vi "Задание_АБ_система ask.vi"() -> ()   [LabVIEW 2017]
uses:
  <vilib>/Analysis/baseanly.llb/Mean (DBL).vi
  <vilib>/gmath/statdist.llb/Normal Random.vi
  <vilib>/Analysis/3filter.llb/Bessel Filter (DBL).vi
  <vilib>/Analysis/NI_AALBase.lvlib
  <vilib>/gmath/NI_Gmath.lvlib
panel:
  out "subarray":dbl[](array[numeric])
  out "Декодированное сообщение 2":dbl[](array[numeric])
  out "x*y 2":i32
  out "x*y":i32
  out "size(s) 2":i32[](array[numeric])
  out "Размер окна с паузами":i32
  out "size(s)":i32
  out "output array":dbl[](array[numeric])
  out "Декодированное сообщение":dbl[](array[numeric])
  in  "Кол-во копий":i32=5
  out "Подготовленный к отправке мажоритарный код":dbl[][](array[numeric])
  out "0, 1":i16[](array[numeric])
  in  "Пороговое значение 2":dbl
  out "Среднее значение":dbl[](array[numeric])
  out "Шум на основе распределения Рэлея":dbl[](graph)
  out "Демодулированный и отфильтрованный сигнал":dbl[](graph)
  in  "Нижняя частота среза":dbl
  in  "Порядок фильтра":i64(slide) scale=0.0..20.0
  in  "Переменная floor(x/y)":i32
  out "Модулирующий сигнал":dbl[](graph)
  out "Частотно модулированный цифровой сигнал":dbl[](graph)
  in  "см. 1.2 Циклов в секунду":i32(slide) scale=4.0..50.0
  in  "Сколько битов брать":i32=4
  out "Радио сигнал с паузами":dbl[](graph)
  in  "Кол-во выборок":i32=400
  out "Массив с паузами":dbl[](array[numeric])
  in  "Количество бит":i32=8
  out "Вырезка из массива":dbl[](array[numeric])
  out "Биты на выходе 1":dbl[](array[numeric])
  # "Демодуляция"
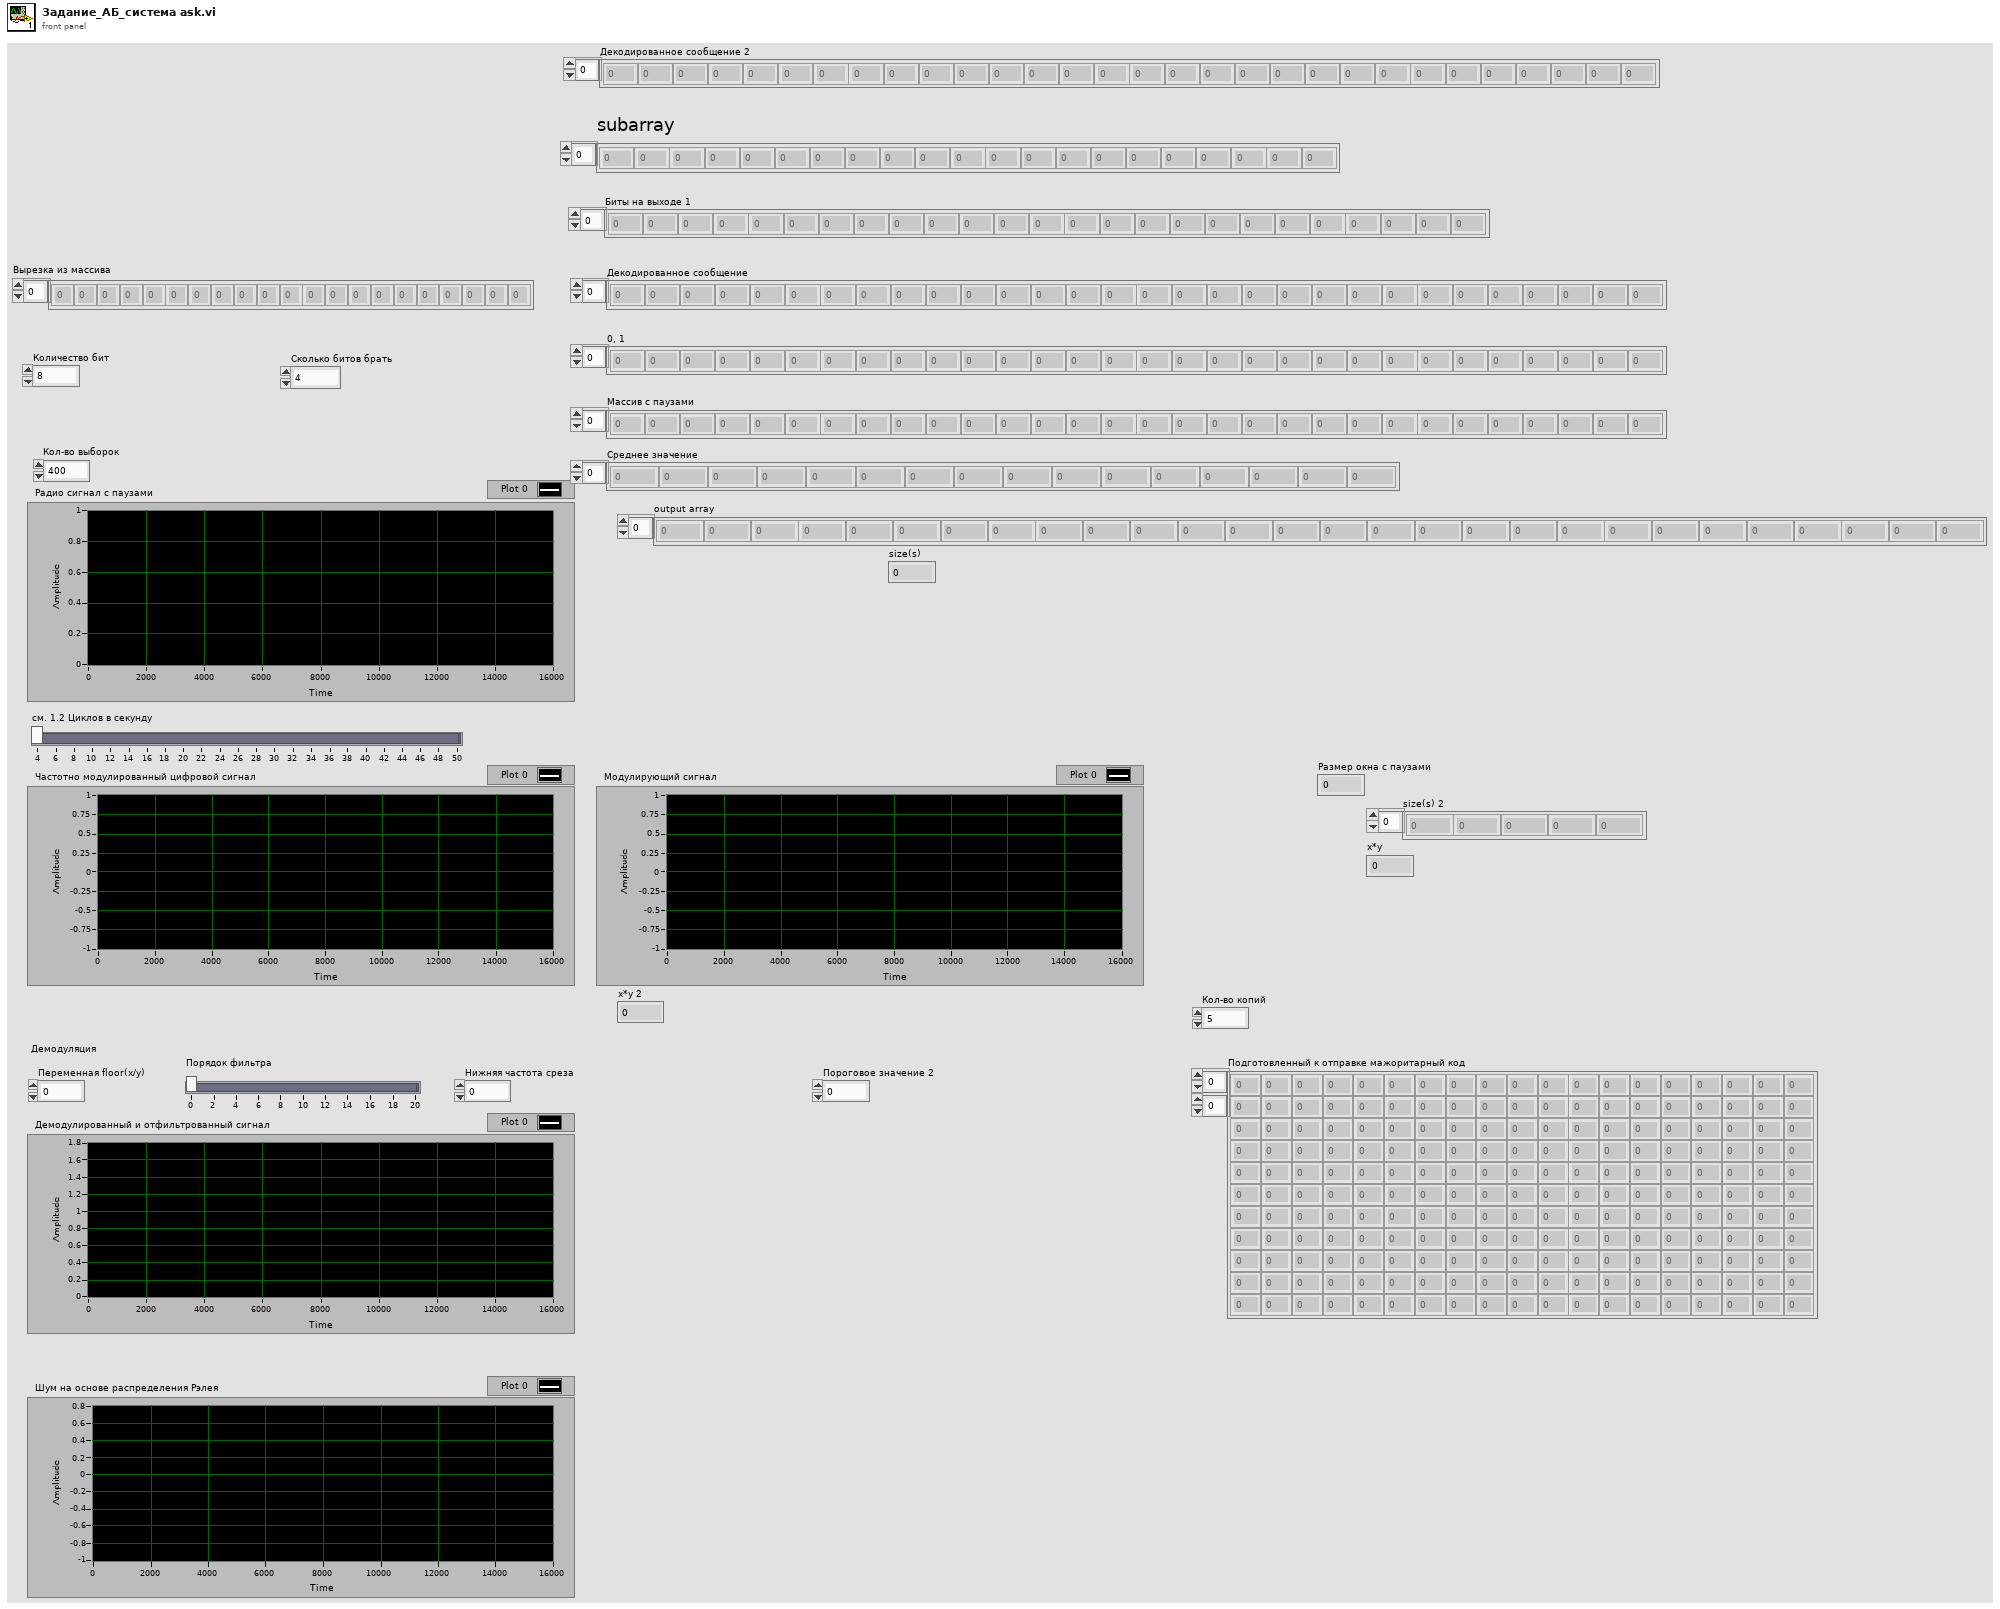
[diagram p1: front panel]
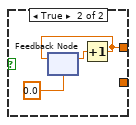
[diagram p3: hidden frame]
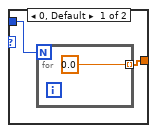
[diagram p4: hidden frame]
diagram:
  w77 = 0  # Начальный бит
  # "Удаление паузы"
  # "Удаление паузы"
  # "(или Декодер? не знаю как правильно назвать)"
  # "Дешифратор мажоритарного когда"
  # "Одномерный из канала"
  # "Получение огибающей"
  # "Регистрация сигнала"
  # "Преобразование в 1 мерный массив модуляции"
  # "п. 1.1 Количество элементов в массиве делим на  размер окна\nполучаем число циклов работы шифратора\n\nп1.2 Вырезаем из последовательности массив с размером окна \nи передаем через shift register\n\nп1.3 Из последовательности вырезаем массив размером с окно и \nдальше передаем на вход системы копирования окна.\n \nп.1.4  В этом пункте мы суммируем предыдущее значение строки со\nстарым для сдвига по длине массива.\n\nп.1.5 Инициализация пустого массива\n\nп.1.6 Создание двухмерного массива из выранных частей предыдущих\nпунктов."
  # "см. 1.1"
  # "Шифратор мажоритарного кода"
  # "1.1 Для модуляции нужно сгенерировать синус \nс количесвом выборок равному количеству \nвыборок в модулирумом сигнале\nПосле локальной переменной !Вырезка из массива! \nЗабираем количество битов с паузами \nУмножаем на два так как после каждого бита добавляется пауза\nи умножаем на Количесво выборок для дальнейшого создания  \nмодулирующего сигнала\n1.2 Циклов в секунду прямой перевод из примера Pulse Demo \nв Examples Finder."
  # "Преобразование двоичной последовательности в радио сигнал"
  # "Частотное модулирование цифрового радио сигнала"
  # "Добавление паузы после каждого бита"
  # "Выборка из последовательности определенного количесва битов"
  # "Генерация случайной последовательности единиц и нулей"
  n1 = for {
    N: "Количество бит" -> [_]
    tunnel: [w79] -> w75 mode=indexing
    n2 = Random Number (0-1)() -> (number: 0 to 1=w84:dbl)
    n3 = Greater Or Equal?(x=w84, y=0.5) -> (x >= y?=w82:bool)
    n4 = Select(t=1.0, s=w82, f=0.0) -> (s? t:f=w79:dbl)
  }
  "Биты на выходе 1" <- w75
  n5 = disable-structure shown="Disabled" {
    frame Disabled {
      n6 = for {
        tunnel: [w85] -> _ mode=indexing
        n7 = feedback #1(0.0) -> (w87:dbl)
        n8 = Increment(x=w87) -> (x+1=w85:dbl)
        n9 = feedback-in #1(w85) -> ()
      }
    }
    frame Enabled {
    }
  }
  n10 = Array Subset "Вырезка из массива"(array=w75, index=w77, length="Сколько битов брать") -> (w73:dbl[])
  "Вырезка из массива" <- w73
  n11 = Array Size "Определение количества пауз"(array=w73) -> (size(s)=w74:i32)
  n12 = for {
    N: w74 -> [_]
    tunnel: w73 -> [w90]
    tunnel: [w89] -> w28 mode=concatenating
    i -> [w88]
    w91 = 0.0  # Значение паузы
    n13 = Array Subset(array=w90, index=w88, length=1) -> (w92:dbl[])
    n14 = Build Array (concatenate)(w92, w91) -> (w89:dbl[])
  }
  "Массив с паузами" <- w28
  n15 = Array Size(array=w28) -> (size(s)=w27:i32)
  "Размер окна с паузами" <- w27
  n16 = Array Size(array=w28) -> (size(s)=w48:i32)
  n17 = Divide(x=w48, y=w27) -> (x/y=w47:dbl)
  n18 = Round Toward +Infinity(x=w47) -> (ceil(x): smallest int >= x=w46:dbl)
  n19 = To Long Integer(number=w46) -> (32bit integer=w45:i32)
  n20 = for {
    N: w45 -> [_]
    shift-right: [w103] -> _
    shift-left: w28 -> [w101]
    tunnel: w27 -> [w102]
    shift-right: [w99] -> _
    shift-left: _ -> [w98]
    tunnel: w27 -> [w100]
    tunnel: [w97] -> _ mode=indexing
    tunnel: [w96] -> w26 mode=concatenating
    tunnel: "Кол-во копий" -> [w94]
    w95 = dbl[][] []  # см. 1.5
    n21 = Split 1D Array "см. 1.2"(array=w101, index=w102) -> (second subarray=w103:dbl[])  [unwired: 1 out]
    n22 = Add "см. 1.4"(x=w100, y=w98) -> (x+y=w99:i32)
    n23 = Array Subset "см. 1.3"(array=w101, length=w100) -> (w97:dbl[])  [unwired: 1 in]
    n24 = for "Копирование окна" {
      N: w94 -> [_]
      tunnel: w97 -> [w105]
      shift-right: [w106] -> w96
      shift-left: w95 -> [w104]
      n25 = Build Array (concatenate) "см. 1.6"(w104, w105) -> (w106:dbl[][])
    }
  }
  "Подготовленный к отправке мажоритарный код" <- w26
  n26 = local read "Размер окна с паузами"() -> (w43:i32)
  n27 = Array Size(array=w26) -> (size(s)=→"size(s) 2":i32[])
  n28 = local read "Кол-во копий"() -> (w42:i32)
  n29 = Multiply(x=w43, y=w42) -> (x*y=w41:i32)
  "x*y" <- w41
  n30 = Reshape Array(w26, w41) -> (w2:dbl[])
  "output array" <- w2
  n31 = Array Size(array=w2) -> (size(s)=→"size(s)":i32)
  n32 = Array Size(array=w2) -> (size(s)=w71:i32)
  n33 = for {
    N: w71 -> [_]
    tunnel: [w109] -> w70 mode=concatenating
    tunnel: w2 -> [w107] mode=indexing
    w112 = 1.0
    # "Кол-во выборок в радио сигнале"
    n34 = Equal?(x=w112, y=w107) -> (x = y?=w113:bool)
    n35 = Select(t=w112, s=w113, f=0.0) -> (s? t:f=w110:dbl)
    n36 = case shown="1" w110 {
      tunnel: [w114 w118] -> w109
      tunnel: "Кол-во выборок" -> [w115 w117]
      frame 0, Default {
        n37 = for {
          N: w115 -> [_]
          tunnel: [0.0] -> w114 mode=indexing
        }
      }
      frame 1 {
        n38 = call <vilib>:"Pulse Pattern.vi"("width"=w117, "delay"=0, "samples"=w117) -> ("Pulse Pattern"=w118:dbl[])  [unwired: 1 in, 1 out]
      }
    }
  }
  "Радио сигнал с паузами" <- w70
  n39 = Array Size(array=w70) -> (size(s)=w72:i32)
  n40 = for {
    N: w72 -> [_]
    tunnel: w70 -> [w128]
    tunnel: [w127] -> w55
    n41 = local read "Размер окна с паузами"() -> (w122:i32)
    n42 = local read "Кол-во копий"() -> (w121:i32)
    n43 = local read "Кол-во выборок"() -> (w125:i32)
    n44 = Multiply(x=w121, y=w122) -> (x*y=w120:i32)
    n45 = Multiply(x=w120, y=w125) -> (x*y=w124:i32)
    n46 = Quotient & Remainder(x=w124, y="см. 1.2 Циклов в секунду") -> (floor(x/y)=w123:i32)  [unwired: 1 out]
    n47 = local write "Переменная floor(x/y)"(w123) -> ()
    n48 = call <vilib>:"Sine Pattern.vi"("cycles"=w123, "samples"=w124) -> ("Sinusoidal Pattern"=w126:dbl[])  [unwired: 2 in, 1 out]
    "Модулирующий сигнал" <- w126
    n49 = Multiply(x=w128, y=w126) -> (x*y=w127:dbl[])
  }
  "Частотно модулированный цифровой сигнал" <- w55
  n50 = local read "Размер окна с паузами"() -> (w57:i32)
  n51 = local read "Кол-во выборок"() -> (w22:i32)
  n52 = local read "Кол-во копий"() -> (w58:i32)
  n53 = Multiply(x=w58, y=w57) -> (x*y=w24:i32)
  n54 = Multiply(x=w24, y=w22) -> (x*y=w23:i32)
  "x*y 2" <- w23
  n55 = call-poly <vilib>:"Continuous Random.vi"("std"=0.2 ("b"), "mean"=0.01 ("x"), "samples"=w23) -> ("normal random data"=w56:dbl[])  [unwired: 7 in, 1 out]
  "Шум на основе распределения Рэлея" <- w56
  n56 = Add(x=w55, y=w56) -> (x+y=w54:dbl[])
  n57 = call-poly <vilib>:"Mean.vi"("X"=w56) -> ()  [unwired: 2 out]
  n58 = local read "Размер окна с паузами"() -> (w61:i32)
  n59 = local read "Кол-во копий"() -> (w19:i32)
  n60 = local read "Кол-во выборок"() -> (w62:i32)
  n61 = Multiply(x=w62, y=w61) -> (x*y=w21:i32)
  n62 = Multiply(x=w21, y=w19) -> (x*y=w20:i32)
  n63 = call <vilib>:"Sine Pattern.vi"("cycles"="Переменная floor(x/y)", "amplitude"=2.0, "samples"=w20) -> ("Sinusoidal Pattern"=w63:dbl[])  [unwired: 1 in, 1 out]
  n64 = Multiply(x=w54, y=w63) -> (x*y=w67:dbl[])
  n65 = Absolute Value(x=w67) -> (abs(x)=w64:dbl[])
  n66 = call-poly <vilib>:"Bessel Filter.vi"("order"="Порядок фильтра", "low cutoff freq: fl"="Нижняя частота среза", "X"=w64) -> ("Filtered X"=w52:dbl[])  [unwired: 5 in, 1 out]
  "Демодулированный и отфильтрованный сигнал" <- w52
  n67 = local read "Кол-во выборок"() -> (w51:i32)
  n68 = Array Size(array=w52) -> (size(s)=w53:i32)
  n69 = Divide(x=w53, y=w51) -> (x/y=w30:dbl)
  n70 = for {
    N: w30 -> [_]
    tunnel: w51 -> [w131]
    shift-right: [w138] -> _
    shift-left: w52 -> [w137]
    tunnel: w51 -> [w134]
    shift-right: [w135] -> _
    shift-left: _ -> [w136]
    tunnel: [w130] -> w1 mode=indexing
    n71 = Split 1D Array(array=w137, index=w131) -> (second subarray=w138:dbl[])  [unwired: 1 out]
    n72 = Array Subset(array=w137, length=w134) -> (w133:dbl[])  [unwired: 1 in]
    n73 = Add(x=w134, y=w136) -> (x+y=w135:i32)
    n74 = Add Array Elements(numeric array=w133) -> (sum=w132:dbl)
    n75 = Divide(x=w132, y=w131) -> (x/y=w130:dbl)
  }
  "Среднее значение" <- w1
  n76 = Greater?(x=w1, y="Пороговое значение 2") -> (0:w49:bool[])
  n77 = Boolean To (0,1)(Boolean=w49) -> (0, 1=→"0, 1":i16[])
  n78 = local read "Размер окна с паузами"() -> (w31:i32)
  n79 = local read "Кол-во копий"() -> (w18:i32)
  n80 = for {
    N: w18 -> [_]
    shift-right: [w145] -> _
    shift-left: w1 -> [w143]
    tunnel: w31 -> [w144]
    shift-right: [w141] -> _
    shift-left: _ -> [w140]
    tunnel: w31 -> [w142]
    tunnel: [w139] -> w32 mode=indexing
    n81 = Split 1D Array "см. 1.2"(array=w143, index=w144) -> (second subarray=w145:dbl[])  [unwired: 1 out]
    n82 = Add "см. 1.4"(x=w142, y=w140) -> (x+y=w141:i32)
    n83 = Array Subset "см. 1.3"(array=w143, length=w142) -> (w139:dbl[])  [unwired: 1 in]
  }
  n84 = local read "Кол-во копий"() -> (w33:i32)
  n85 = Array Size(array=w32) -> (size(s)=w40:i32[])
  n86 = Index Array "см. 2.1"(array=w40, index #1=0 ("index"), index #2=1 ("index")) -> (element #1=w37:i32, element #2=w36:i32)
  n87 = Divide(x=w37, y=w33) -> (x/y=w35:dbl)
  n88 = To Long Integer(number=w35) -> (32bit integer=w34:i32)
  n89 = Multiply(x=w34, y=w36) -> (x*y=w17:i32)
  n90 = for {
    N: w17 -> [_]
    tunnel: w32 -> [w181]
    tunnel: w36 -> [w173]
    tunnel: w33 -> [w166]
    tunnel: [w161] -> w11 mode=indexing
    tunnel: [w149] -> w5 mode=indexing
    w180 = 1  # кол-во столбцов
    w171 = 0  # Строка
    # "Разделение по элементам"
    # "Кажется тут я перепутал названия  \nПотом сделаю правильно"
    # "Счетчик строк см 2.3"
    # "Счетчик столбцов см. 2.2"
    n91 = feedback #2(0) -> (w169:dbl)
    n92 = Equal?(x=w173, y=w169) -> (x = y?=w175:bool)
    n93 = Select(t=0.0, s=w175, f=w169) -> (s? t:f=w168:dbl)
    n94 = Increment(x=w168) -> (x+1=w167:dbl)
    n95 = feedback-in #2(w167) -> ()
    n96 = Wait (ms)(milliseconds to wait=u32 0) -> ()  [unwired: 1 out]
    n97 = Select(t=w166, s=w175, f=w171) -> (s? t:f=w172:i32)
    n98 = feedback #3(0) -> (w174:i32)
    n99 = Add(x=w172, y=w174) -> (x+y=w170:i32)
    n100 = feedback-in #3(w170) -> ()
    n101 = Array Subset "см. 2.4"(array=w181, index (row)=w170, length (row)=w166, index (col)=w168, length (col)=w180) -> (w182:dbl[][])
    n102 = Reshape Array "см. 2.5"(w182, w166) -> (w146:dbl[])
    n103 = Array Size(array=w146) -> (size(s)=w165:i32)
    n104 = for {
      N: w165 -> [_]
      tunnel: w146 -> [w193] mode=indexing
      tunnel: [w188] -> w160
      tunnel: [w184] -> w159
      n105 = Greater Or Equal?(x=w193, y=0.5) -> (x >= y?=w194:bool)
      n106 = case shown="False" w194 {
        tunnel: [_ w199] -> w192
        tunnel: [w196 _] -> w191
        frame False {
          n107 = feedback #4(0.0) -> (w197:dbl)
          n108 = Increment(x=w197) -> (x+1=w196:dbl)
          n109 = feedback-in #4(w196) -> ()
        }
        frame True {
          n110 = feedback #5(0.0) -> (w200:dbl)
          n111 = Increment(x=w200) -> (x+1=w199:dbl)
          n112 = feedback-in #5(w199) -> ()
        }
      }
      n113 = feedback #6(0.0) -> (w183:dbl)
      n114 = Greater?(x=w191, y=w183) -> (0:w190:bool)
      n115 = Select(t=w191, s=w190, f=w183) -> (s? t:f=w188:dbl)
      n116 = feedback-in #6(w188) -> ()
      n117 = feedback #7(0.0) -> (w186:dbl)
      n118 = Greater?(x=w192, y=w186) -> (0:w187:bool)
      n119 = Select(t=w192, s=w187, f=w186) -> (s? t:f=w184:dbl)
      n120 = feedback-in #7(w184) -> ()
    }
    n121 = Round To Nearest(number=w146) -> (nearest integer value=w150:dbl[])
    n122 = Equal?(x=1, y=w150) -> (x = y?=w152:bool[])
    n123 = Boolean To (0,1)(Boolean=w152) -> (0, 1=w148:i16[])
    n124 = Not(x=w152) -> (.not. x?=w153:bool[])
    n125 = Boolean To (0,1)(Boolean=w153) -> (0, 1=w147:i16[])
    n126 = Add Array Elements(numeric array=w148) -> (sum=w155:i16)
    n127 = Add Array Elements(numeric array=w147) -> (sum=w154:i16)
    n128 = Greater?(x=w155, y=w154) -> (0:w158:bool)
    n129 = Greater?(x=w159, y=w160) -> (0:w164:bool)
    n130 = Select(t=1.0, s=w164, f=0.0) -> (s? t:f=w161:dbl)
    n131 = Select(t=1.0, s=w158, f=0.0) -> (s? t:f=w149:dbl)
  }
  "Декодированное сообщение" <- w11
  "Декодированное сообщение 2" <- w5
  n132 = Array Size(array=w11) -> (size(s)=w14:i32)
  n133 = for {
    N: w14 -> [_]
    tunnel: w11 -> [w206]
    tunnel: [w203] -> w16 mode=indexing
    i -> [w204]
    n134 = Multiply(x=2, y=w204) -> (x*y=w202:i32)
    n135 = Index Array(array=w206, index=w202) -> (element=w203:dbl)
  }
  n136 = Array Size(array=w5) -> (size(s)=w8:i32)
  n137 = for {
    N: w8 -> [_]
    tunnel: w5 -> [w211]
    tunnel: [w208] -> w10 mode=indexing
    i -> [w209]
    n138 = Multiply(x=2, y=w209) -> (x*y=w207:i32)
    n139 = Index Array(array=w211, index=w207) -> (element=w208:dbl)
  }
  n140 = Divide(x=w14, y=2) -> (x/y=w12:dbl)
  n141 = Array Subset(array=w16, index=0, length=w12) -> ()  [unwired: 1 out]
  n142 = Divide(x=w8, y=2) -> (x/y=w6:dbl)
  n143 = Array Subset(array=w10, index=0, length=w6) -> (→"subarray":dbl[])
